vi "Read Tag All.vi"(6 "error in (no error)":errorcluster, 10 "Tag.lvclass":refnum<class "Tag.lvclass">) -> (0 "TagPreviousY":dbl, 1 "TagPreviousX":dbl, 2 "TagY":dbl, 3 "TagX":dbl, 4 "error out":errorcluster, 5 "Tag ID":dbl)   [LabVIEW 2014, in "Tag.lvclass"]
uses:
  Tag.lvclass
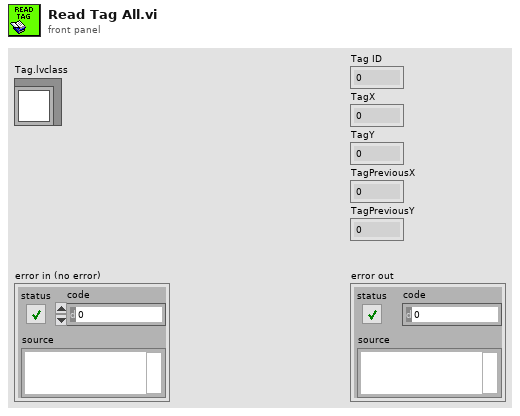
[diagram p1: front panel]
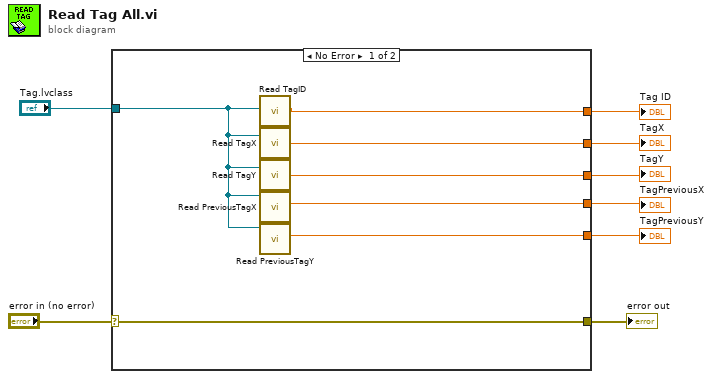
[diagram p0: block diagram]
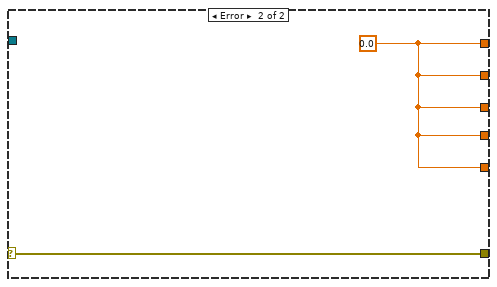
[diagram p2: hidden frame]
diagram:
  n1 = case shown="No Error" "error in (no error)" {
    selector: "error in (no error)" -> [w15 w16]
    tunnel: [w15 w16] -> w7
    tunnel: "Tag.lvclass" -> [w10 _]
    tunnel: [w9 w17] -> w5
    tunnel: [w14 w17] -> w4
    tunnel: [w13 w17] -> w3
    tunnel: [w12 w17] -> w2
    tunnel: [w11 w17] -> w1
    frame No Error {
      n2 = call "Read TagID.vi"("Tag in"=w10) -> ("TagID"=w9:dbl)  [unwired: 16 in, 2 out]
      n3 = call-dynamic "Read TagX.vi"("Tag in"=w10) -> ("RealTagX"=w14:dbl)  [unwired: 1 in, 2 out]
      n4 = call-dynamic "Read TagY.vi"("Tag in"=w10) -> ("RealTagY"=w13:dbl)  [unwired: 1 in, 2 out]
      n5 = call-dynamic "Read PreviousTagX.vi"("Tag in"=w10) -> ("PreviousTagX"=w12:dbl)  [unwired: 8 in, 2 out]
      n6 = call-dynamic "Read PreviousTagY.vi"("Tag in"=w10) -> ("PreviousTagY"=w11:dbl)  [unwired: 8 in, 2 out]
    }
    frame Error {
      w17 = 0.0 ("TagID")
    }
  }
  "error out" <- w7
  "Tag ID" <- w5
  "TagX" <- w4
  "TagY" <- w3
  "TagPreviousX" <- w2
  "TagPreviousY" <- w1
